vi "Prep Controller.vi"(6 "Interlock Q Class out":refnum<class "Interlock Q Class.lvclass">, 8 "error in (no error)":errorcluster, 9 "Laser State Data":refnum<data-value>, 10 "Process State Data":refnum<data-value>, 11 "Laser Controller in":refnum<class "Laser Controller.lvclass">) -> (0 "error out":errorcluster, 3 "Laser Controller out":refnum<class "Laser Controller.lvclass">)   [LabVIEW 2022 SP3, in "Laser Controller.lvclass"]
uses:
  Laser Controller.lvclass
  XY Stage/Process Actor/Process Framework/Interlock Q Class/Interlock Q Class.lvclass
  XY Stage/Process Actor/Process Framework/Process State Data/Process State Data.lvclass
  Laser State Data/Laser State Data.lvclass
  Laser Controller.lvclass/Laser Controller.ctl
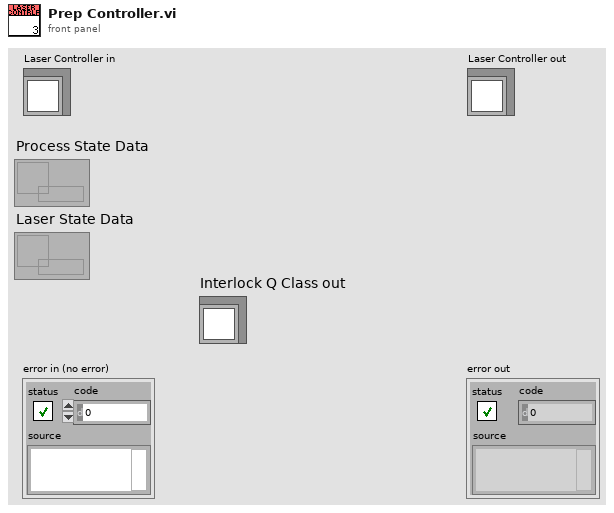
[diagram p1: front panel]
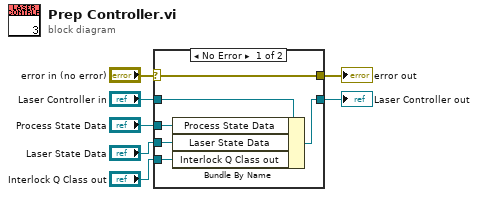
[diagram p0: block diagram]
diagram:
  n1 = case shown="No Error" "error in (no error)" {
    selector: "error in (no error)" -> [w12 w15]
    tunnel: [w12 w15] -> w6
    tunnel: [w11 w14] -> w4
    tunnel: "Laser Controller in" -> [w13 w14]
    tunnel: "Laser State Data" -> [w10 _]
    tunnel: "Process State Data" -> [w9 _]
    tunnel: "Interlock Q Class out" -> [w8 _]
    frame No Error {
      n2 = Bundle By Name(cluster=w13, "Process State Data"=w9, "Laser State Data"=w10, "Interlock Q Class out"=w8) -> (w11:refnum<class "Laser Controller.lvclass">)
    }
    frame Error {
    }
  }
  "error out" <- w6
  "Laser Controller out" <- w4
